vi "Open.vi"(8 "error in":errorcluster, 9 "Timeout":i32=2000 format="%.0f ms", 11 "Reply Protocol in":refnum<class "Reply Protocol DataSocket.lvclass">) -> (0 "error out":errorcluster, 3 "Reply Protocol out":refnum<class "Reply Protocol DataSocket.lvclass">)   [LabVIEW 2023, in "HAL GOOP4.lvlib" / "Reply Protocol DataSocket.lvclass"]
uses:
  Reply Protocol DataSocket.lvclass
  Reply Protocol DataSocket.lvclass/Reply Protocol DataSocket.ctl
  Reply Protocol Base/Reply Protocol Base.lvclass/Reply Protocol Base.ctl
  Reply Protocol Base/Reply Protocol Base.lvclass
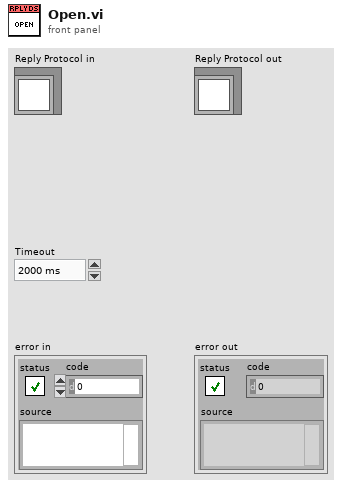
[diagram p1: front panel]
types:
  T1 = enum16{"Read", "Write", "ReadWrite", "BufferedRead", "BufferedReadWrite"}
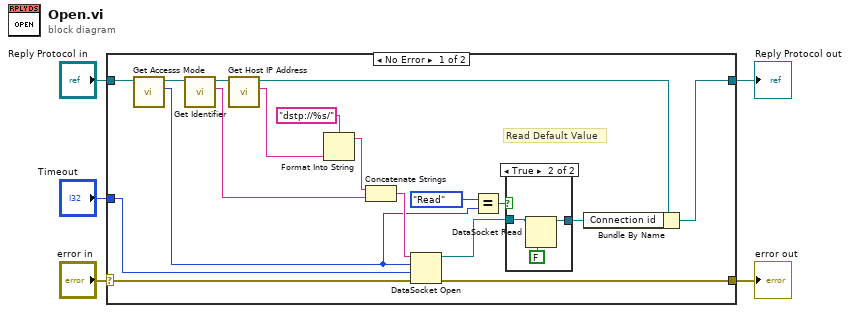
[diagram p0: block diagram]
diagram:
  n1 = case shown="No Error" "error in" {
    selector: "error in" -> [w23 w29]
    tunnel: [w16 w29] -> w5
    tunnel: [w19 w28] -> w4
    tunnel: "Reply Protocol in" -> [w21 w28]
    tunnel: "Timeout" -> [w20 _]
    frame No Error {
      # "Read Default Value"
      n2 = call "Get Accesss Mode.vi"("Reply Protocol DataSocket in"=w21) -> ("Accesss Mode"=w8:T1, "Reply Protocol DataSocket out"=w11:refnum<class "Reply Protocol DataSocket.lvclass">)  [unwired: 9 in]
      n3 = call "Get Identifier.vi"("Reply Protocol Base in"=w11) -> ("Identifier"=w17:string, "Reply Protocol Base out"=w18:refnum<class "Reply Protocol DataSocket.lvclass">)  [unwired: 9 in]
      n4 = call "Get Host IP Address.vi"("Reply Protocol DataSocket in"=w18) -> ("Host IP Address"=w13:string, "Reply Protocol DataSocket out"=w14:refnum<class "Reply Protocol DataSocket.lvclass">)  [unwired: 9 in]
      n5 = Format Into String(format string="dstp://%s/", w13) -> (resulting string=w12:string)  [unwired: 2 in, 1 out]
      n6 = Concatenate Strings(w12, w17) -> (w22:string)
      n7 = DataSocket Open(8:w23, 9:w20, 10:w8, 11:w22) -> (0:w16:errorcluster, 3:w7:refnum<k13>)
      n8 = Equal?(x=T1."Read" ("mode"), y=w8) -> (x = y?=w10:bool)
      n9 = case shown="True" w10 {
        tunnel: w7 -> [w24 w27]
        tunnel: [w24 w26] -> w6
        frame False {
        }
        frame True {
          n10 = DataSocket Read(6:FALSE ("wait for updated value (T)"), 11:w27) -> (3:w26:refnum<k13>)  [unwired: 3 in, 6 out]
        }
      }
      n11 = Bundle By Name(cluster=w14, "Connection id"=w6) -> (w19:refnum<class "Reply Protocol DataSocket.lvclass">)
    }
    frame Error {
    }
  }
  "error out" <- w5
  "Reply Protocol out" <- w4
